vi "drivetrain_ftsec_to_raw.vi"(11 "Drive Data":cluster{"Left":dbl, "Right":dbl}) -> (3 "Drive Data Out":cluster{"Left":dbl, "Right":dbl})   [LabVIEW 2011]
uses:
  gear_shift_state.ctl
  drivetrain_globals.vi
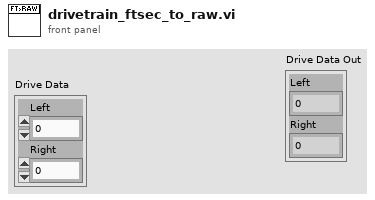
[diagram p1: front panel]
types:
  T1 = typedef "gear_shift_state.ctl" = enum16{"low", "high"}
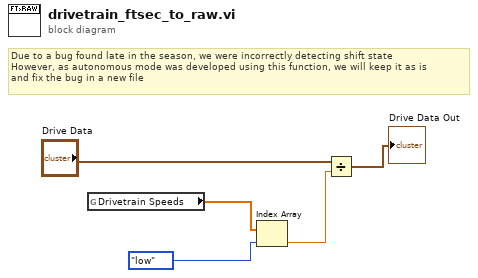
[diagram p0: block diagram]
diagram:
  # "Due to a bug found late in the season, we were incorrectly detecting shift state\nHowever, as autonomous mode was developed using this function, we will keep it as is\nand fix the bug in a new file"
  n1 = global read "drivetrain_globals.vi" "Drivetrain Speeds"() -> (w5:dbl[])
  n2 = Index Array(array=w5, index=gear_shift_state."low" ("gear shift state")) -> (element=w2:dbl)
  n3 = Divide(x="Drive Data", y=w2) -> (x/y=→"Drive Data Out":cluster{"Left":dbl, "Right":dbl})
